vi "CRYChange Name by Step Editor.vi"(8 "New Names Type":string[](array[string]), 9 "Old Names Type":string[](array[string]), 10 "Old Names":string[](array[string]), 11 "New Names":string[](array[string])) -> ()   [LabVIEW 2013]
uses:
  CRYMainGlobal.vi
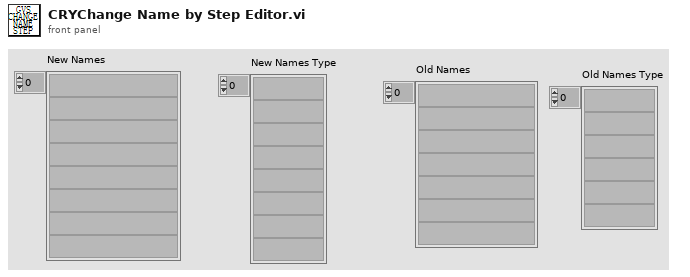
[diagram p1: front panel]
types:
  T1 = typedef "CRYStep.ctl" = cluster{"No.VI":i32, "Category":string, "StepName":string, "Seq setup flattened":string, "Comment":string, "Steps config.":bool[], "Jump config":i32[], "Start":dbl, "Increment":dbl, "Name":string, "Unit":string, "Y data":u16, "Y prefix":string, "Y dB ref":dbl, "Y unit":string, "Repeat State Array":cluster{"Start":dbl, "Increment":dbl, "Count":i32, "Num":i32}[]}
  T2 = typedef "CRYChanged Names Cluster.ctl" = cluster{"Input Channel":T3, "Output Channel":T3, "Cuve":T3, "Value":T3, "Result":T3, "Wave":T3}
  T3 = typedef "CRYChanged Data Array Cluster.ctl" = cluster{"Rename":T4[], "Delete":T4[]}
  T4 = typedef "CRYChanged Data Cluster.ctl" = cluster{"Old Name":string, "New Name":string}
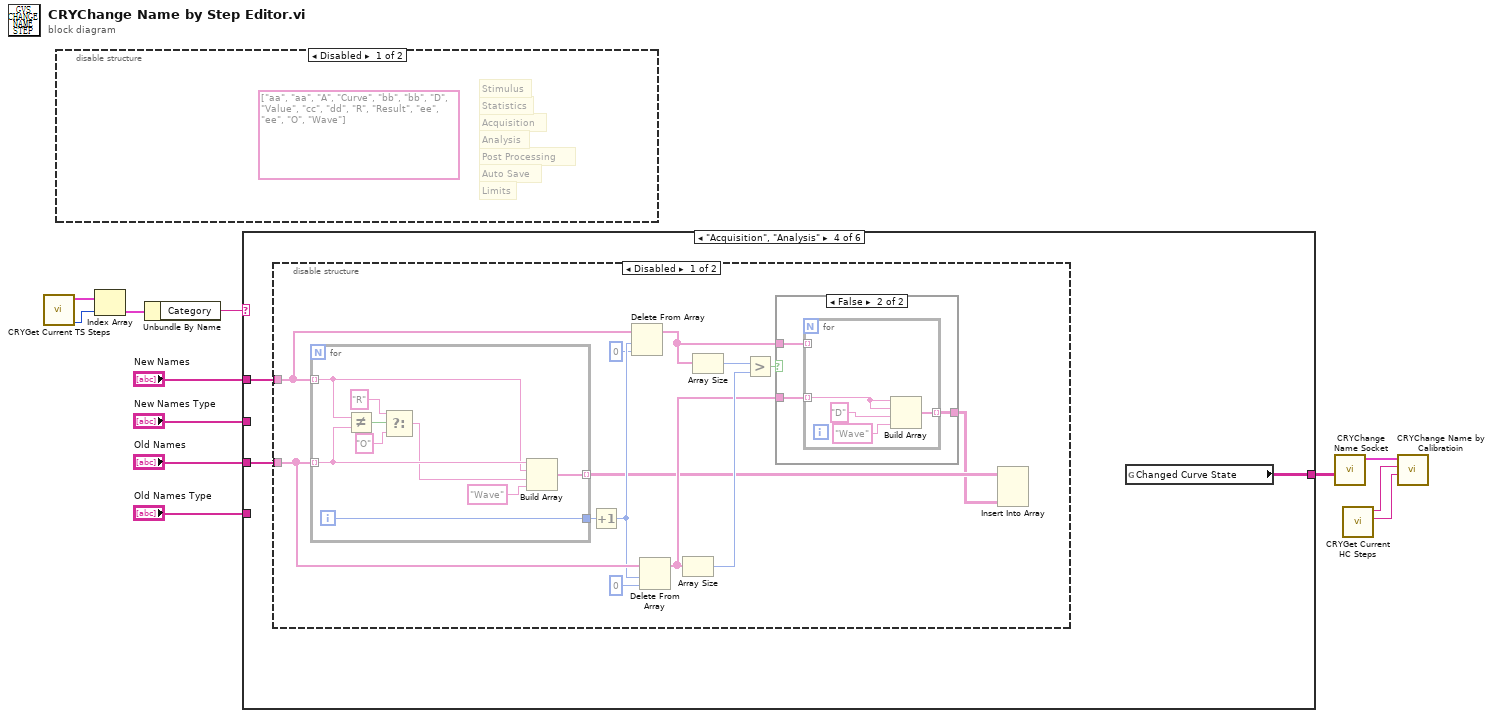
[diagram p0: block diagram]
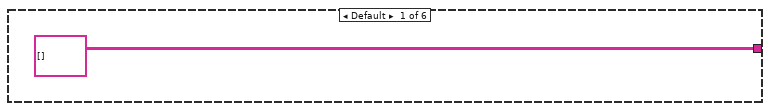
[diagram p3: hidden frame]
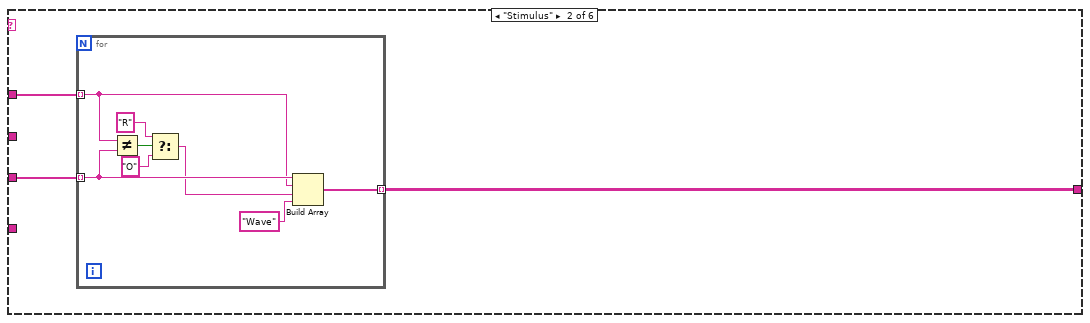
[diagram p4: hidden frame]
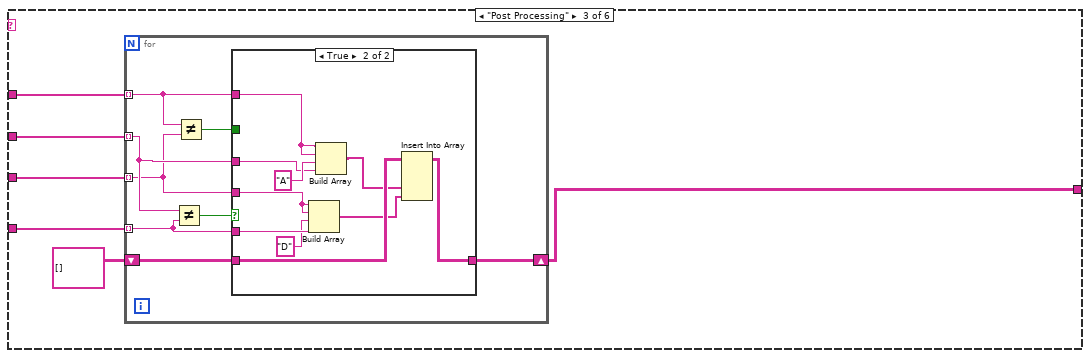
[diagram p5: hidden frame]
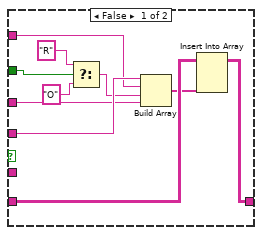
[diagram p6: hidden frame]
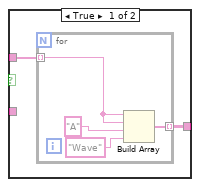
[diagram p7: hidden frame]
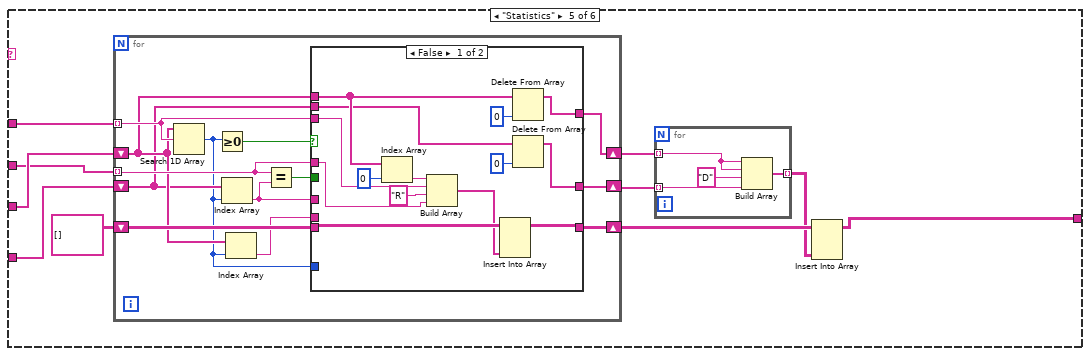
[diagram p9: hidden frame]
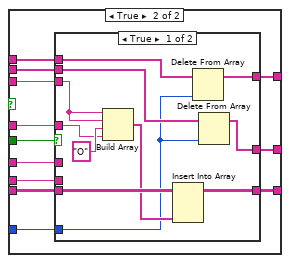
[diagram p10: hidden frame]
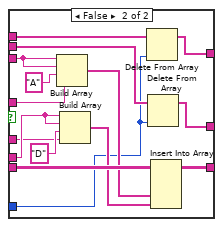
[diagram p11: hidden frame]
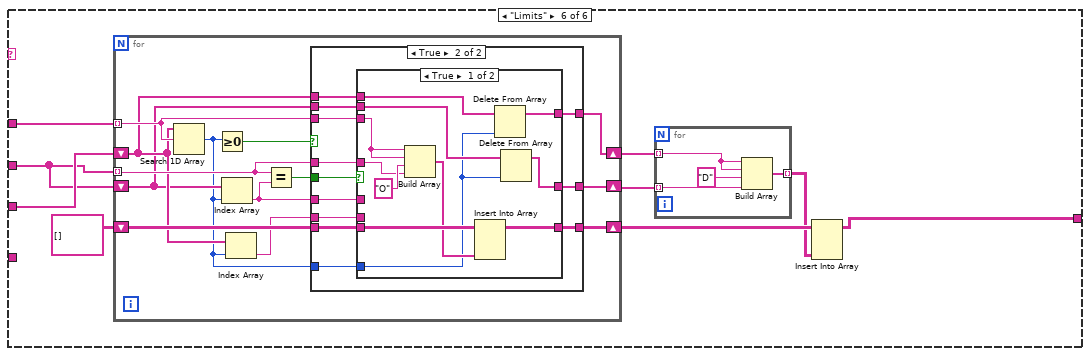
[diagram p12: hidden frame]
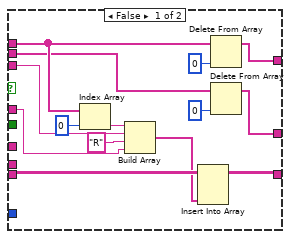
[diagram p13: hidden frame]
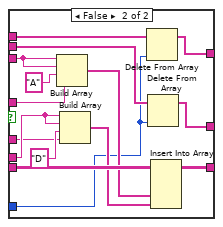
[diagram p14: hidden frame]
diagram:
  n1 = call "CRYGet Current TS Steps.vi"() -> ("SelectStepNumber in Tree"=w8:i32, "Steps"=w9:T1[])  [unwired: 1 in, 9 out]
  n2 = disable-structure shown="Disabled" {
    frame Disabled {
      (unwired) string[][] [["aa", "aa", "A", "Curve"], ["bb", "bb", "D", "Value"], ["cc", "dd", "R", "Result"], ["ee", "ee", "O", "Wave"]] ("Calibration Data In")
      # "Auto Save"
      # "Limits"
      # "Post Processing"
      # "Analysis"
      # "Acquisition"
      # "Stimulus"
      # "Statistics"
    }
    frame Enabled {
    }
  }
  n3 = Index Array(array=w9, index=w8) -> (element=w7:T1)
  n4 = Unbundle By Name(w7) -> ("Category"=w6:string)
  n5 = case shown="\"Acquisition\", \"Analysis\"" w6 {
    tunnel: "Old Names" -> [_ w16 w30 w60 w105 w183]
    tunnel: "New Names" -> [_ w15 w29 w61 w106 w184]
    tunnel: [string[][] [] w14 w25 w59 w97 w177] -> w10
    tunnel: "Old Names Type" -> [_ _ w27 _ w104 _]
    tunnel: "New Names Type" -> [_ _ w28 _ w103 w176]
    frame Default {
    }
    frame "Stimulus" {
      n6 = for {
        tunnel: w16 -> [w23] mode=indexing
        tunnel: w15 -> [w19] mode=indexing
        tunnel: [w17] -> w14 mode=indexing
        n7 = Not Equal?(x=w19, y=w23) -> (x != y?=w22:bool)
        n8 = Select(t="R" ("String"), s=w22, f="O") -> (s? t:f=w18:string)
        n9 = Build Array(w23, w19, w18, "Wave" ("element")) -> (w17:string[])
      }
    }
    frame "Post Processing" {
      n10 = for {
        tunnel: w30 -> [w35] mode=indexing
        tunnel: w29 -> [w36] mode=indexing
        tunnel: w28 -> [w37] mode=indexing
        tunnel: w27 -> [w34] mode=indexing
        shift-right: [w32] -> w25
        shift-left: string[][] [] -> [w33]
        n11 = Not Equal?(x=w37, y=w34) -> (x != y?=w38:bool)
        n12 = Not Equal?(x=w36, y=w35) -> (x != y?=w31:bool)
        n13 = case shown="True" w38 {
          tunnel: w37 -> [w46 w51]
          tunnel: w36 -> [w47 w54]
          tunnel: w35 -> [w48 w58]
          tunnel: w34 -> [_ w50]
          tunnel: w33 -> [w41 w57]
          tunnel: [w39 w55] -> w32
          tunnel: w31 -> [w43 _]
          frame False {
            n14 = Select(t="R" ("String"), s=w43, f="O") -> (s? t:f=w42:string)
            n15 = Build Array(w48, w47, w42, w46) -> (w40:string[])
            n16 = Insert Into Array(array=w41, new element=w40) -> (w39:string[][])  [unwired: 2 in]
          }
          frame True {
            n17 = Build Array(w58, w58, "D" ("element"), w50) -> (w56:string[])
            n18 = Build Array(w54, w54, "A" ("element"), w51) -> (w53:string[])
            n19 = Insert Into Array(array=w57, new element #1=w53, new element #2=w56) -> (w55:string[][])  [unwired: 2 in]
          }
        }
      }
    }
    frame "Acquisition", "Analysis" {
      n20 = disable-structure shown="Disabled" {
        disable-tunnel: w61 -> [w73 _]
        disable-tunnel: w60 -> [w71 _]
        frame Disabled {
          n21 = for {
            tunnel: w71 -> [w95] mode=indexing
            tunnel: w73 -> [w91] mode=indexing
            tunnel: [w89] -> w64 mode=indexing
            tunnel: [w88] -> w72
            i -> [w88]
            n22 = Not Equal?(x=w91, y=w95) -> (x != y?=w94:bool)
            n23 = Select(t="R" ("String"), s=w94, f="O") -> (s? t:f=w90:string)
            n24 = Build Array(w95, w91, w90, "Wave" ("element")) -> (w89:string[])
          }
          n25 = Increment(x=w72) -> (x+1=w70:i32)
          n26 = Delete From Array(array=w73, length=w70, index=0) -> (array with subset deleted=w66:string[])  [unwired: 1 out]
          n27 = Delete From Array(array=w71, length=w70, index=0) -> (array with subset deleted=w65:string[])  [unwired: 1 out]
          n28 = Array Size(array=w65) -> (size(s)=w67:i32)
          n29 = Array Size(array=w66) -> (size(s)=w62:i32)
          n30 = Greater?(x=w62, y=w67) -> (0:w74:bool)
          n31 = case shown="False" w74 {
            tunnel: w66 -> [w76 w83]
            tunnel: [w75 w82] -> w63
            tunnel: w65 -> [_ w81]
            frame True {
              n32 = for {
                tunnel: w76 -> [w78] mode=indexing
                tunnel: [w77] -> w75 mode=indexing
                n33 = Build Array(w78, w78, "A" ("String"), "Wave" ("element")) -> (w77:string[])
              }
            }
            frame False {
              n34 = for {
                tunnel: w83 -> [_] mode=indexing
                tunnel: [w85] -> w82 mode=indexing
                tunnel: w81 -> [w84] mode=indexing
                n35 = Build Array(w84, w84, "D" ("String"), "Wave" ("element")) -> (w85:string[])
              }
            }
          }
          n36 = Insert Into Array(array=w64, new element=w63) -> ()  [unwired: 2 in, 1 out]
        }
        frame Enabled {
        }
      }
      n37 = global read "CRYMainGlobal.vi" "Changed Curve State"() -> (w59:string[][])
    }
    frame "Statistics" {
      n38 = for {
        tunnel: w106 -> [w122] mode=indexing
        tunnel: w103 -> [w121] mode=indexing
        shift-right: [w120] -> w99
        shift-left: string[][] [] -> [w119]
        shift-right: [w112] -> w101
        shift-left: w105 -> [w115]
        shift-right: [w111] -> w100
        shift-left: w104 -> [w114]
        n39 = Search 1D Array(1D array=w115, element=w122) -> (index of element=w113:i32)  [unwired: 1 in]
        n40 = Greater Or Equal To 0?(x=w113) -> (x >= 0?=w123:bool)
        n41 = Index Array(array=w114, index=w113) -> (element=w116:string)
        n42 = Index Array(array=w115, index=w113) -> (element=w117:string)
        n43 = Equal?(x=w121, y=w116) -> (x = y?=w118:bool)
        n44 = case shown="False" w123 {
          tunnel: w122 -> [w136 w149]
          tunnel: w121 -> [w124 w148]
          tunnel: [w132 w146] -> w120
          tunnel: w119 -> [w133 w147]
          tunnel: w118 -> [_ w145]
          tunnel: w117 -> [_ w144]
          tunnel: w116 -> [_ w143]
          tunnel: w115 -> [w130 w142]
          tunnel: w114 -> [w126 w141]
          tunnel: w113 -> [_ w140]
          tunnel: [w128 w139] -> w112
          tunnel: [w125 w138] -> w111
          frame False {
            n45 = Index Array(array=w130, index=0) -> (element=w135:string)
            n46 = Build Array(w135, w136, "R" ("f"), w124) -> (w131:string[])
            n47 = Insert Into Array(array=w133, new element=w131) -> (w132:string[][])  [unwired: 2 in]
            n48 = Delete From Array(array=w130, index=0) -> (array with subset deleted=w128:string[])  [unwired: 1 in, 1 out]
            n49 = Delete From Array(array=w126, index=0) -> (array with subset deleted=w125:string[])  [unwired: 1 in, 1 out]
          }
          frame True {
            n50 = case shown="True" w145 {
              tunnel: w149 -> [w160 w175]
              tunnel: w148 -> [w155 w166]
              tunnel: w147 -> [w159 w174]
              tunnel: [w157 w172] -> w146
              tunnel: w144 -> [_ w170]
              tunnel: w143 -> [_ w168]
              tunnel: w142 -> [w154 w165]
              tunnel: w141 -> [w153 w164]
              tunnel: w140 -> [w152 w163]
              tunnel: [w151 w162] -> w139
              tunnel: [w150 w161] -> w138
              frame True {
                n51 = Build Array(w160, w160, "O" ("element"), w155) -> (w158:string[])
                n52 = Insert Into Array(array=w159, new element=w158) -> (w157:string[][])  [unwired: 2 in]
                n53 = Delete From Array(array=w154, index=w152) -> (array with subset deleted=w151:string[])  [unwired: 1 in, 1 out]
                n54 = Delete From Array(array=w153, index=w152) -> (array with subset deleted=w150:string[])  [unwired: 1 in, 1 out]
              }
              frame False {
                n55 = Build Array(w175, w175, "A" ("element"), w166) -> (w173:string[])
                n56 = Build Array(w170, w170, "D" ("String"), w168) -> (w171:string[])
                n57 = Delete From Array(array=w165, index=w163) -> (array with subset deleted=w162:string[])  [unwired: 1 in, 1 out]
                n58 = Delete From Array(array=w164, index=w163) -> (array with subset deleted=w161:string[])  [unwired: 1 in, 1 out]
                n59 = Insert Into Array(array=w174, new element #1=w173, new element #2=w171) -> (w172:string[][])  [unwired: 2 in]
              }
            }
          }
        }
      }
      n60 = for {
        tunnel: [w109] -> w98 mode=indexing
        tunnel: w101 -> [w108] mode=indexing
        tunnel: w100 -> [w107] mode=indexing
        n61 = Build Array(w108, w108, "D" ("String"), w107) -> (w109:string[])
      }
      n62 = Insert Into Array(array=w99, new element=w98) -> (w97:string[][])  [unwired: 2 in]
    }
    frame "Limits" {
      n63 = for {
        tunnel: w184 -> [w200] mode=indexing
        tunnel: w176 -> [w199] mode=indexing
        shift-right: [w198] -> w179
        shift-left: string[][] [] -> [w197]
        shift-right: [w190] -> w181
        shift-left: w183 -> [w193]
        shift-right: [w189] -> w180
        shift-left: w176 -> [w192]
        n64 = Search 1D Array(1D array=w193, element=w200) -> (index of element=w191:i32)  [unwired: 1 in]
        n65 = Greater Or Equal To 0?(x=w191) -> (x >= 0?=w201:bool)
        n66 = Index Array(array=w192, index=w191) -> (element=w194:string)
        n67 = Index Array(array=w193, index=w191) -> (element=w195:string)
        n68 = Equal?(x=w199, y=w194) -> (x = y?=w196:bool)
        n69 = case shown="True" w201 {
          tunnel: w200 -> [w214 w227]
          tunnel: w199 -> [w202 w226]
          tunnel: [w210 w224] -> w198
          tunnel: w197 -> [w211 w225]
          tunnel: w196 -> [_ w223]
          tunnel: w195 -> [_ w222]
          tunnel: w194 -> [_ w221]
          tunnel: w193 -> [w208 w220]
          tunnel: w192 -> [w204 w219]
          tunnel: w191 -> [_ w218]
          tunnel: [w206 w217] -> w190
          tunnel: [w203 w216] -> w189
          frame False {
            n70 = Index Array(array=w208, index=0) -> (element=w213:string)
            n71 = Build Array(w213, w214, "R" ("f"), w202) -> (w209:string[])
            n72 = Insert Into Array(array=w211, new element=w209) -> (w210:string[][])  [unwired: 2 in]
            n73 = Delete From Array(array=w208, index=0) -> (array with subset deleted=w206:string[])  [unwired: 1 in, 1 out]
            n74 = Delete From Array(array=w204, index=0) -> (array with subset deleted=w203:string[])  [unwired: 1 in, 1 out]
          }
          frame True {
            n75 = case shown="True" w223 {
              tunnel: w227 -> [w238 w253]
              tunnel: w226 -> [w233 w244]
              tunnel: w225 -> [w237 w252]
              tunnel: [w235 w250] -> w224
              tunnel: w222 -> [_ w248]
              tunnel: w221 -> [_ w246]
              tunnel: w220 -> [w232 w243]
              tunnel: w219 -> [w231 w242]
              tunnel: w218 -> [w230 w241]
              tunnel: [w229 w240] -> w217
              tunnel: [w228 w239] -> w216
              frame True {
                n76 = Build Array(w238, w238, "O" ("element"), w233) -> (w236:string[])
                n77 = Insert Into Array(array=w237, new element=w236) -> (w235:string[][])  [unwired: 2 in]
                n78 = Delete From Array(array=w232, index=w230) -> (array with subset deleted=w229:string[])  [unwired: 1 in, 1 out]
                n79 = Delete From Array(array=w231, index=w230) -> (array with subset deleted=w228:string[])  [unwired: 1 in, 1 out]
              }
              frame False {
                n80 = Build Array(w253, w253, "A" ("element"), w244) -> (w251:string[])
                n81 = Build Array(w248, w248, "D" ("String"), w246) -> (w249:string[])
                n82 = Delete From Array(array=w243, index=w241) -> (array with subset deleted=w240:string[])  [unwired: 1 in, 1 out]
                n83 = Delete From Array(array=w242, index=w241) -> (array with subset deleted=w239:string[])  [unwired: 1 in, 1 out]
                n84 = Insert Into Array(array=w252, new element #1=w251, new element #2=w249) -> (w250:string[][])  [unwired: 2 in]
              }
            }
          }
        }
      }
      n85 = for {
        tunnel: [w187] -> w178 mode=indexing
        tunnel: w181 -> [w186] mode=indexing
        tunnel: w180 -> [w185] mode=indexing
        n86 = Build Array(w186, w186, "D" ("String"), w185) -> (w187:string[])
      }
      n87 = Insert Into Array(array=w179, new element=w178) -> (w177:string[][])  [unwired: 2 in]
    }
  }
  n88 = call "CRYChange Name Socket.vi"("Data"=w10) -> ("Changed Name"=w12:T2)  [unwired: 10 in]
  n89 = call "CRYGet Current HC Steps.vi"() -> ("Calibration setup flattened Out"=w1:string, "Hardware setup flattened Out"=w2:string)  [unwired: 10 in]
  n90 = call "CRYChange Name by Calibratioin.vi"("Calibration In"=w1, "Hardware In"=w2, "Changed Names"=w12) -> ()  [unwired: 9 in]
